vi "ADAM_Server_Channels.vi"() -> (0 "DAQ Error":errorcluster)   [LabVIEW 2017]
uses:
  ADAM Client/Sub VIs/ADAM Controls/Search_mode.ctl
  <vilib>/Analysis/baseanly.llb/Mean (DBL).vi
  Globals/Meas_global.vi
  Globals/Trav_pos_global.vi
  <vilib>/Analysis/NI_AALBase.lvlib
panel:
  out "Waveform Graph":dbl[][](graph)
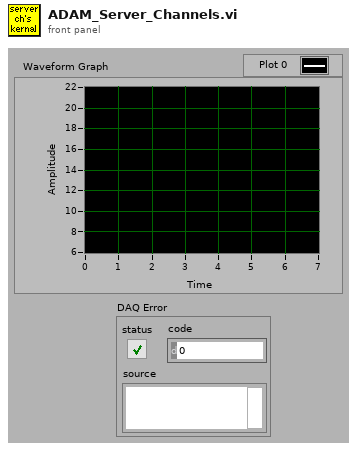
[diagram p1: front panel]
types:
  T1 = typedef "Analysis_info_cluster.ctl" = cluster{"Colour":u32, "Inst type":T2, "Inst name":string, "Symbol":string, "Code name":string, "Extra Info":string, "Inst Array":T3, "Extra Titles":string[], "Extra Values":string[], "U":dbl, "u^2":dbl, "u^3":dbl, "u^4":dbl, "Skew_u":dbl, "Kurt_u":dbl, "Sd Error in Mean":dbl, "% u'/U":dbl, "X":dbl, "Y":dbl, "Z":dbl, "Timescale integral Estimate":dbl, "Sd Error in Variance":dbl, "Calib File":path, "Calib Constants":dbl[], "Output Position":bool, "Full Stats":bool, "Av Sampling Rate":dbl, "Av No of Samples":dbl, "Total Meas Time (s)":dbl, "ADAM Ch Name":string, "Max value":dbl, "Min value":dbl, "Sync Delay Time (s)":dbl}
  T2 = typedef "Inst_type.ctl" = enum16{"Propeller anemometer", "Raw voltage", "Pressure Transducer", "Pitot-static tube", "Preston tube", "Hot wire", "Cross wire 1", "Cross wire 2", "Generic Linear", "Generic Polynomial", "Generic BackPoly", "Fast FID", "Thermocouple", "Cold wire", "Pulsed Wire", "LDA Vel", "LDA Tran time", "LDA Arr time", "Microphone"}
  T3 = typedef "Instrument_Array.ctl" = enum16{"PWA", "LDA", "Analogue"}
  T4 = typedef "Search_mode.ctl" = enum16{"Between times", "All Times"}
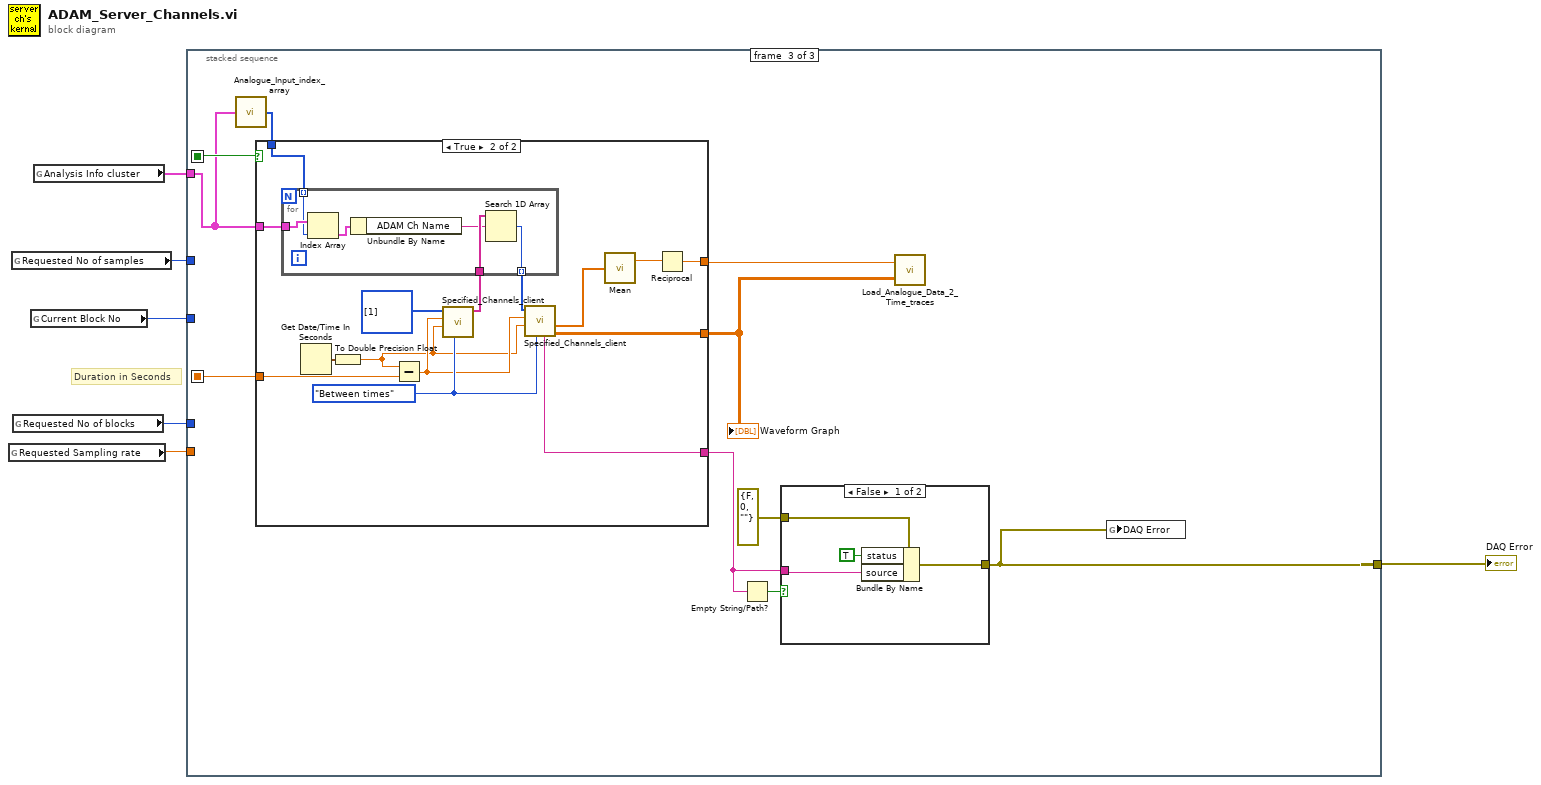
[diagram p0: block diagram]
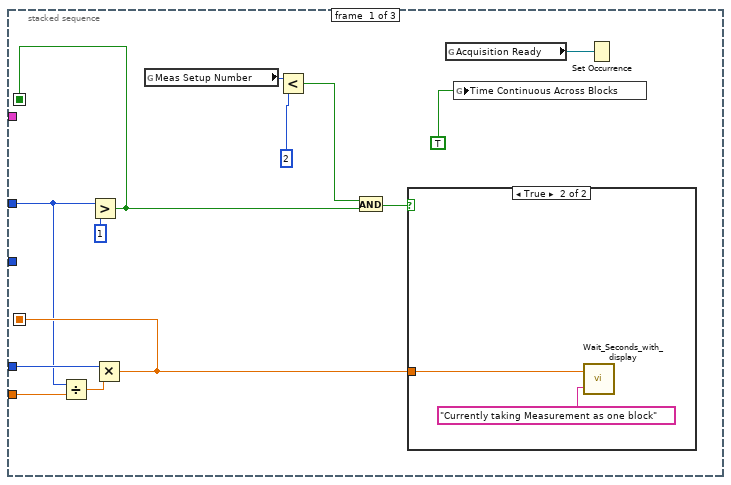
[diagram p2: hidden frame]
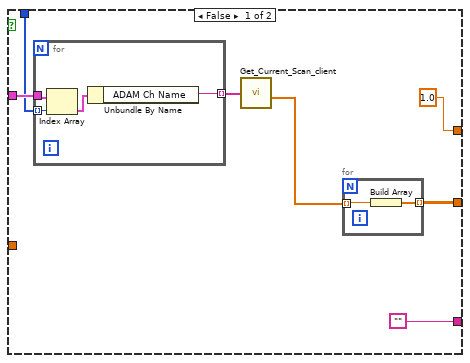
[diagram p5: hidden frame]
diagram:
  # "Duration in Seconds"
  n1 = global read "Meas_global.vi" "Requested Sampling rate"() -> (w5:dbl)
  n2 = global read "Meas_global.vi" "Requested No of samples"() -> (w6:i32)
  n3 = global read "Meas_global.vi" "Requested No of blocks"() -> (w2:i32)
  n4 = global read "Meas_global.vi" "Current Block No"() -> (w4:i32)
  n5 = global read "Meas_global.vi" "Analysis Info cluster"() -> (w3:T1[])
  n6 = stacked-sequence {
    seq-local: [w16 _ _] -> [_ _ w31]
    seq-local: [w10 _ _] -> [_ _ w27]
    tunnel: w6 -> [w15 _ _]
    tunnel: w4 -> [_ _ _]
    tunnel: w3 -> [_ _ w25]
    tunnel: w5 -> [w19 _ _]
    tunnel: w2 -> [w17 _ _]
    tunnel: [_ _ w26] -> w1
    frame #0 {
      n7 = Divide(x=w15, y=w19) -> (x/y=w18:dbl)
      n8 = Greater?(x=w15, y=1) -> (0:w10:bool)
      n9 = Multiply(x=w17, y=w18) -> (x*y=w16:dbl)
      n10 = global read "Trav_pos_global.vi" "Meas Setup Number"() -> (w13:i32)
      n11 = Less?(x=w13, y=2) -> (x < y?=w11:bool)
      n12 = And(x=w11, y=w10) -> (x .and. y?=w9:bool)
      n13 = case shown="True" w9 {
        tunnel: w16 -> [_ w20]
        frame False {
        }
        frame True {
          n14 = call "Wait_Seconds_with_display.vi"("Message"="Currently taking Measurement as one block", "Seconds to wait"=w20) -> ()  [unwired: 2 out]
        }
      }
      n15 = global read "Meas_global.vi" "Acquisition Ready"() -> (w7:refnum<k4>)
      n16 = global write "Meas_global.vi" "Time Continuous Across Blocks"(TRUE ("Time Continuous across Blocks")) -> ()
      n17 = Set Occurrence(w7) -> ()
    }
    frame #1 {
    }
    frame #2 {
      n18 = call "Analogue_Input_index_array.vi"("Analysis Info cluster"=w25) -> ("Array"=w24:i32[])
      n19 = case shown="True" w27 {
        tunnel: w31 -> [_ w58]
        tunnel: [w35 w53] -> w23
        tunnel: w25 -> [w38 w52]
        tunnel: [1.0 w50] -> w22
        tunnel: ["" w49] -> w28
        tunnel: w24 -> [w32 w45]
        frame False {
          n20 = for {
            tunnel: w38 -> [w43]
            tunnel: [w44] -> w37 mode=indexing
            tunnel: w32 -> [w41] mode=indexing
            n21 = Index Array(array=w43, index=w41) -> (element=w42:T1)
            n22 = Unbundle By Name(w42) -> ("ADAM Ch Name"=w44:string)
          }
          n23 = call "Get_Current_Scan_client.vi"("ADAM Ch Names"=w37) -> ("Numerical Values"=w36:dbl[])  [unwired: 1 in, 2 out]
          n24 = for {
            tunnel: w36 -> [w40] mode=indexing
            tunnel: [w39] -> w35 mode=indexing
            n25 = Build Array(w40) -> (w39:dbl[])
          }
        }
        frame True {
          w54 = Search_mode."Between times" ("Mode")
          n26 = Get Date/Time In Seconds() -> (seconds since 1Jan1904=w59:timestamp)
          n27 = To Double Precision Float(number=w59) -> (double precision float=w47:dbl)
          n28 = Subtract(x=w47, y=w58) -> (x-y=w48:dbl)
          n29 = call "Specified_Channels_client.vi"("Mode"=w54, "End time"=w47, "Start time"=w48, "ADAM Index array"=i32[] [1]) -> ("All Active Ch Names"=w56:string[])  [unwired: 1 in, 6 out]
          n30 = for {
            tunnel: w52 -> [w62]
            tunnel: w56 -> [w65]
            tunnel: [w64] -> w55 mode=indexing
            tunnel: w45 -> [w60] mode=indexing
            n31 = Index Array(array=w62, index=w60) -> (element=w61:T1)
            n32 = Unbundle By Name(w61) -> ("ADAM Ch Name"=w63:string)
            n33 = Search 1D Array(1D array=w65, element=w63) -> (index of element=w64:i32)  [unwired: 1 out]
          }
          n34 = call "Specified_Channels_client.vi"("Mode"=w54, "End time"=w47, "Start time"=w48, "ADAM Index array"=w55) -> ("Output array"=w53:dbl[][], "Averaging Period"=w46:dbl[], "Messages"=w49:string)  [unwired: 1 in, 4 out]
          n35 = call-poly <vilib>:"Mean.vi"("X"=w46) -> ("mean"=w51:dbl)  [unwired: 1 out]
          n36 = Reciprocal(x=w51) -> (1/x=w50:dbl)
        }
      }
      "Waveform Graph" <- w23
      n37 = Empty String/Path?(string/path=w28) -> (empty?=w30:bool)
      n38 = case shown="False" w30 {
        tunnel: errorcluster {"status"=FALSE, "code"=0, "source"=""} ("DAQ Error") -> [w69 w70]
        tunnel: [w68 w70] -> w26
        tunnel: w28 -> [w66 _]
        frame False {
          n39 = Bundle By Name(cluster=w69, "status"=TRUE, "source"=w66) -> (w68:errorcluster)
        }
        frame True {
        }
      }
      n40 = call "Load_Analogue_Data_2_Time_traces.vi"("Voltage Array"=w23, "Sampling Rate (Hz)"=w22) -> ()  [unwired: 1 in]
      n41 = global write "Meas_global.vi" "DAQ Error"(w26) -> ()
    }
  }
  "DAQ Error" <- w1
